vi "Main.vi"() -> ()   [LabVIEW 2016]
uses:
  Type Definitions/Fisher Paykel Motor Profile.ctl
  Type Definitions/FisherPaykel Direction CMD.ctl
  Type Definitions/Fisher Paykel Feedback Commands.ctl
  Type Definitions/Fisher Paykel Agitate Parameters.ctl
  Type Definitions/FisherPaykel Set Sense Profile.ctl
  Type Definitions/Fisher Paykel Friction Profile.ctl
  Type Definitions/Fisher Paykel Bridge Test Profile.ctl
  Trunk/Utility/LabVIEW GEA2 Toolkit v1.0.0.0/type defs/ERD Read Data In.ctl
  Trunk/Utility/LabVIEW GEA2 Toolkit v1.0.0.0/type defs/Data Type.ctl
  Trunk/Washer HCC/Washer HCC NEWFI/Type Definitions/HCC Washer Types.ctl
  Type Definitions/Fisher Paykel Spin PID.ctl
  Trunk/Utility/LabVIEW GEA2 Toolkit v1.0.0.0/type defs/Source_Destination.ctl
  Trunk/Utility/LabVIEW GEA2 Toolkit v1.0.0.0/type defs/Data Out.ctl
  Type Definitions/Fisher Paykel Main Command.ctl
  Trunk/Utility/Save File/File Setup (Public)/Type Definition/Save File DOE LabView Program.ctl
  <vilib>/Utility/file.llb/Write Delimited Spreadsheet (string).vi
  C:/TechLab/NI-2010/Trunk/Utility/LabVIEW GEA2 Toolkit v1.0.0.0/Appliance.NET/GeaCommunication.dll
  Trunk/Utility/LabVIEW GEA2 Toolkit v1.0.0.0/Appliance.NET/GeaCommunication.dll
  Trunk/Utility/LabVIEW GEA2 Toolkit v1.0.0.0/library/GEA2_Toolkit.lvlib
  Trunk/Utility/Save File/File Setup.lvlib
panel:
  out "Exit App":bool
  out "Start DAQ Loop":bool
  in  "OK":bool
  in  "Read ERD List (2017) 2":T1[](array[typedef])=[{"ERD Number"=61623, "Data Type"=enum."string"}, {"ERD Number"=61617, "Data Type"=enum."string"}, {"ERD Number"=65314, "Data Type"=enum."string"}, {"ERD Number"=61563, "Data Type"=enum."string"}, {"ERD Number"=61537, "Data Type"=enum."uint32_t"}, {"ERD Number"=61612, "Data Type"=enum."string"}] {"ERD Number" format="%.0x"}
  out "File  Version":string="Parametric Stand"
  in  "Error In":errorcluster
  out "Error Out":errorcluster
  in  "Tab Control":T3(tab)
  in  "Set Motor Number":bool
  in  "Motor Number":u16=130 max=255 step=1
  in  "Bridge Test Profile":bool
  in  "Move with Bridge Test Profile":T4
  in  "Test Friction Profile":bool
  in  "Move With Friction Test Profile":T5
  in  "Set Sense Profile":bool
  in  "Set Sense Profile":T6
  in  "Move With Stepper Profile":bool
  in  "Reset Fault Flags":bool
  in  "Set Current Limit":bool
  out "Feedback Command Read":string
  out "Agitate Profile Command Read":string
  in  "Send Command":bool
  in  "Stop Motor (Spin)":bool
  in  "Start Agitate Profile":bool
  in  "Agitate Parameters":T7={"Agitate Running Time (sec)"=15, "Direction (CW or CCW)"="1", "RampUpTime (1-600ms)"=250, "TargetSpeed (0-200RPM)"=726, "PlateauTime (0-1800ms 10ms Increment)"=1000, "PauseTime (0-1800ms 10ms Increment)"=600} {"PauseTime (0-1800ms 10ms Increment)" step=10; "PlateauTime (0-1800ms 10ms Increment)" step=10; "TargetSpeed (0-200RPM)" max=1600 step=1; "RampUpTime (1-600ms)" max=600 step=10; "Agitate Running Time (sec)" step=1}
  in  "Start Spin Profile":bool
  out "Spin Profile Command Read":string
  in  "Spin Profile":T9={"Target Speed (RPM)"=23, "Acceleration Rate - (10 Slowest/1000 Fastest)"=10, "Running Time (s)"=0, "Direction (CW or CCW)"="0"} {"Running Time (s)" step=1; "Acceleration Rate - (10 Slowest/1000 Fastest)" min=10 max=1000 step=1; "Target Speed (RPM)" min=23 max=1600 step=1}
  in  "Stop Motor (Agitate)":bool
  in  "Feedback Commands":T10
  in  "Current Limit - (1-50) - (0.1-5A)":u16 max=50 step=1
  in  "Spin PID":T11={"Kp"=1.84, "Ki"=0.03, "Kd"=0.0, "Kc"=0.06} {"Kc" min=0.0 max=1.0; "Kd" min=0.0 max=1.0; "Ki" min=0.0 max=1.0; "Kp" min=0.0 max=16.0}
  in  "Agitate PID":T11={"Kp"=1.84, "Ki"=0.03, "Kd"=0.0, "Kc"=0.06} {"Kc" min=0.0 max=1.0; "Kd" min=0.0 max=1.0; "Ki" min=0.0 max=1.0; "Kp" min=0.0 max=16.0}
  in  "Spin CMD Speed (mS)":u32=150
  in  "Agitate CMD Speed (mS)":u32=150
  in  "Record":bool
  out "File Path":path
  in  "Read Inverter ERDs":bool
  in  "Read Machine ERDs":bool
  out "ERD Array":string[][](array[string])=[["Motor Profile Status (0xF0B7)", "Started"], ["Motor Profile (0xF0B7)", "9"], ["Motor Mode (0xF0B1)", "Idle"], ["Mode Shift Status (0xFF22)", "Agitate State"], ["Sub-Cycle (0xF07B)", "WASH"], ["Remaining Cycle Time(s) (0xF061)", "1707"], ["Target Speed (RPM) (0xF0AC)", "0"], ["Basket Speed (RPM) (0xF0A9)", ""]]
  in  "Read ERD List (2017)":T1[](array[typedef])=[{"ERD Number"=61623, "Data Type"=enum."string"}, {"ERD Number"=61617, "Data Type"=enum."string"}, {"ERD Number"=65314, "Data Type"=enum."string"}, {"ERD Number"=61563, "Data Type"=enum."string"}, {"ERD Number"=61537, "Data Type"=enum."uint32_t"}, {"ERD Number"=61612, "Data Type"=enum."string"}, {"ERD Number"=61609, "Data Type"=enum."uint16_t"}, {"ERD Number"=62218, "Data Type"=enum."string"}, {"ERD Number"=62229, "Data Type"=enum."string"}, {"ERD Number"=62224, "Data Type"=enum."string"}] {"ERD Number" format="%.0x"}
  in  "Run With Machine Controls":bool
  in  "Enable Diagnostic Data":T12=enum."2017 Washer"
  in  "Agitate Parameters Settle Stroke":T7={"Agitate Running Time (sec)"=15, "Direction (CW or CCW)"="1", "RampUpTime (1-600ms)"=250, "TargetSpeed (0-200RPM)"=683, "PlateauTime (0-1800ms 10ms Increment)"=150, "PauseTime (0-1800ms 10ms Increment)"=600} {"PauseTime (0-1800ms 10ms Increment)" step=10; "PlateauTime (0-1800ms 10ms Increment)" step=10; "TargetSpeed (0-200RPM)" max=1600 step=1; "RampUpTime (1-600ms)" max=600 step=10; "Agitate Running Time (sec)" step=1}
  in  "2019 Inverter CMDs":T1[](array[typedef])=[{"ERD Number"=62218, "Data Type"=enum."string"}, {"ERD Number"=62229, "Data Type"=enum."string"}, {"ERD Number"=62224, "Data Type"=enum."string"}] {"ERD Number" format="%.0x"}
  in  "Disable Serial":bool
  out "Use GEA Inverter Output":bool
  in  "GEA Inputs":T13={"Source"=240, "Destination"=35} {"Destination" format="%.0x"; "Source" format="%.0x"}
  out "Debug array":string[](array[string])
  in  "Turn on Text Debug Array":bool
  in  "Inverter Address":T13={"Source"=240, "Destination"=63} {"Destination" format="%.0x"; "Source" format="%.0x"}
  out "Debug Save Array":string[](array[string])
  # "MOTOR CONTROL INTERFACE"
  # "Start Speed > End Speed"
  # "Agitate Profile Parameters"
  # "Agitate Start Parameters"
  # "Spin Profile Parameters"
  # "Spin Start Parameters"
  # "2017 ERD List\nMotor Profile Status (0xF0B7) - string\nMotor Mode (0xF0B1) - string\nMode Shift Status (0xFF22) - string\nSub-Cycle (0xF07B) - string\nRemaining Cycle Time(s) (0xF061) - U32\nTarget Speed (RPM) (0xF0AC) - string\nBasket Speed (0xF0A9) -U16"
  # "2015 ERD List\nMotor Profile Status (0xF319) - string\nMotor Mode (0xF313) - string\nMode Shift Status (0xF31D) - string\nSub-Cycle (0xF213) - string\nRemaining Cycle Time(s) (0xF140) - U32\nTarget Speed (RPM) (0xF30E) - string\nBasket Speed (0xF30B)-U16"
  # "2019 Inverter ERD List\nPower-W (0xF30A) - string\nDriving Speed-RPM (0xF315)-string\nActual Speed-RPM (0xF310)-string"
  # "Agitate Profile Parameters"
  # "Agitate Start Parameters"
  # "Version 34 - Read Machine ERDs and Read Inverter ERDS unchecked by default"
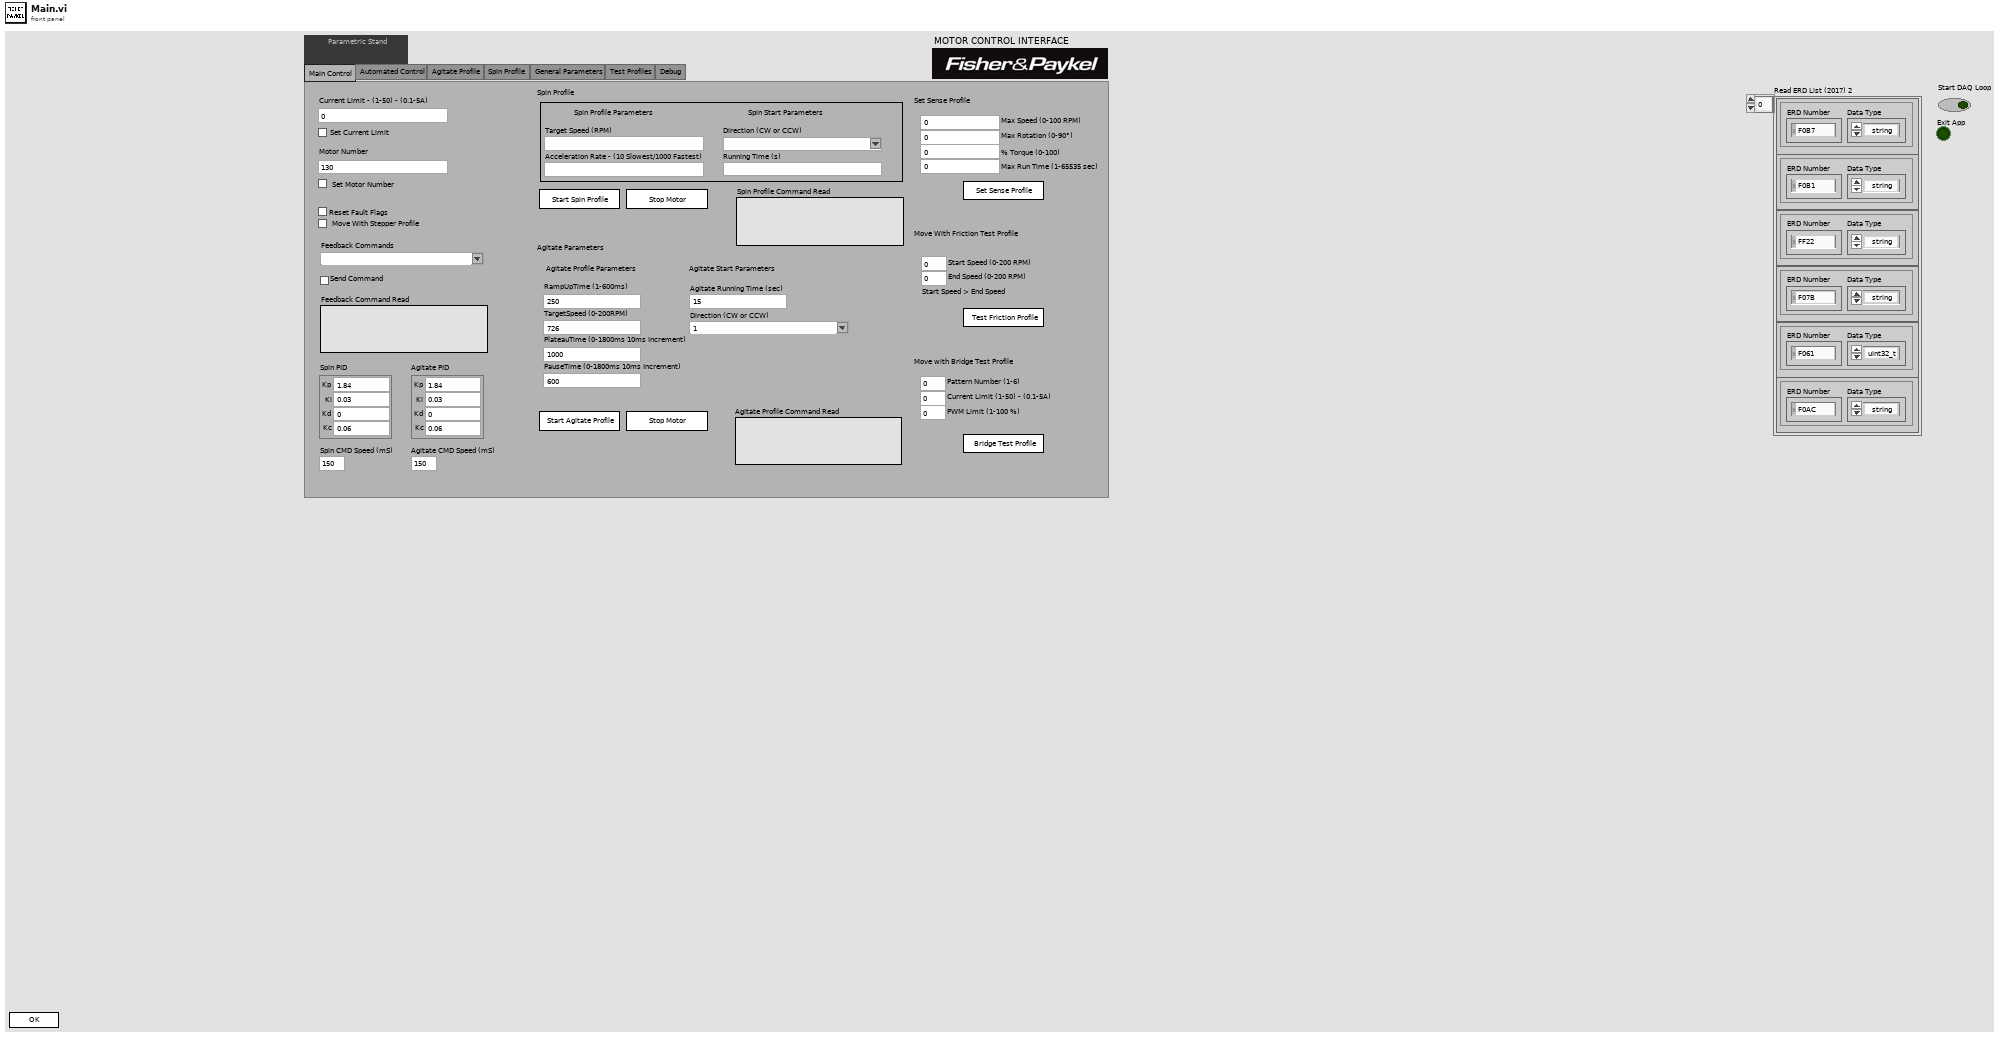
[diagram p1: front panel]
types:
  T1 = typedef "GEA2_Toolkit.lvlib/ERD Read Data In.ctl" = cluster{"ERD Number":u16, "Data Type":T2}
  T2 = typedef "GEA2_Toolkit.lvlib/Data Type.ctl" = enum16{"string", "boolean", "uint8_t", "uint16_t", "uint32_t", "uint64_t"}
  T3 = enum32{"Main Control", "Automated Control", "Agitate Profile", "Spin Profile", "General Parameters", "Test Profiles", "Debug"}
  T4 = typedef "Fisher Paykel Bridge Test Profile.ctl" = cluster{"Pattern Number (1-6)":u16, "Current Limit (1-50) - (0.1-5A)":u16, "PWM Limit (1-100 %)":u16}
  T5 = typedef "Fisher Paykel Friction Profile.ctl" = cluster{"Start Speed (0-200 RPM)":u16, "End Speed (0-200 RPM)":u16}
  T6 = typedef "FisherPaykel Set Sense Profile.ctl" = cluster{"Max Speed (0-100 RPM)":u16, "Max Rotation (0-90°)":u16, "% Torque (0-100)":u16, "Max Run Time (1-65535 sec)":u16}
  T7 = typedef "Fisher Paykel Agitate Parameters.ctl" = cluster{"Agitate Running Time (sec)":u16, "Direction (CW or CCW)":T8, "RampUpTime (1-600ms)":u16, "TargetSpeed (0-200RPM)":u16, "PlateauTime (0-1800ms 10ms Increment)":u16, "PauseTime (0-1800ms 10ms Increment)":u16}
  T8 = typedef "FisherPaykel Direction CMD.ctl" = string
  T9 = typedef "Fisher Paykel Motor Profile.ctl" = cluster{"Target Speed (RPM)":u16, "Acceleration Rate - (10 Slowest/1000 Fastest)":u16, "Running Time (s)":u16, "Direction (CW or CCW)":T8}
  T10 = typedef "Fisher Paykel Feedback Commands.ctl" = string
  T11 = typedef "Fisher Paykel Spin PID.ctl" = cluster{"Kp":dbl, "Ki":dbl, "Kd":dbl, "Kc":dbl}
  T12 = typedef "HCC Washer Types.ctl" = enum16{"", "Viper Washer", "Hawk Washer", "2015 Washer", "2017 Washer"}
  T13 = typedef "GEA2_Toolkit.lvlib/Source_Destination.ctl" = cluster{"Source":u8, "Destination":u8}
  T14 = typedef "Fisher Paykel Main Command.ctl" = string
  T15 = enum32{"invalid app kind", "Development System", "Run Time System", "Student Edition", "Embedded LabVIEW", "Evaluation", "Custom"}
  T16 = enum32{"Invalid", "Standard", "Closed", "Hidden", "Minimized", "Maximized"}
  T17 = typedef "File Setup.lvlib/Save File DOE LabView Program.ctl" = enum16{"No Name Found", "DOE Stand", "Dishwasher Kitchen", "Portable Stand", "HEWH", "Dryer", "Dryer WILT", "HCC", "PRAT", "HEWH RLT", "Refrigeration"}
  T18 = cluster{"Core":cluster{"Current VI Reference":refnum<vi>, "Close Panel on Exit?":bool}, "VISA Output":refnum<visa-resource-name>, "ERD Array":string[][], "Spin Profile":T9, "Agitate Parameters":T7, "GEA Stop Toggle":u8}
  T19 = cluster{"Current VI Reference":refnum<vi>, "Close Panel on Exit?":bool}
  T20 = typedef "FileVersionInformation.ctl" = cluster{"FileVersion":string, "ProductName":string, "InternalName":string, "CompanyName":string, "LegalCopyright":string, "FileDescription":string}
  T21 = enum16{"open", "replace", "create", "open or create", "replace or create", "replace or create with confirmation"}
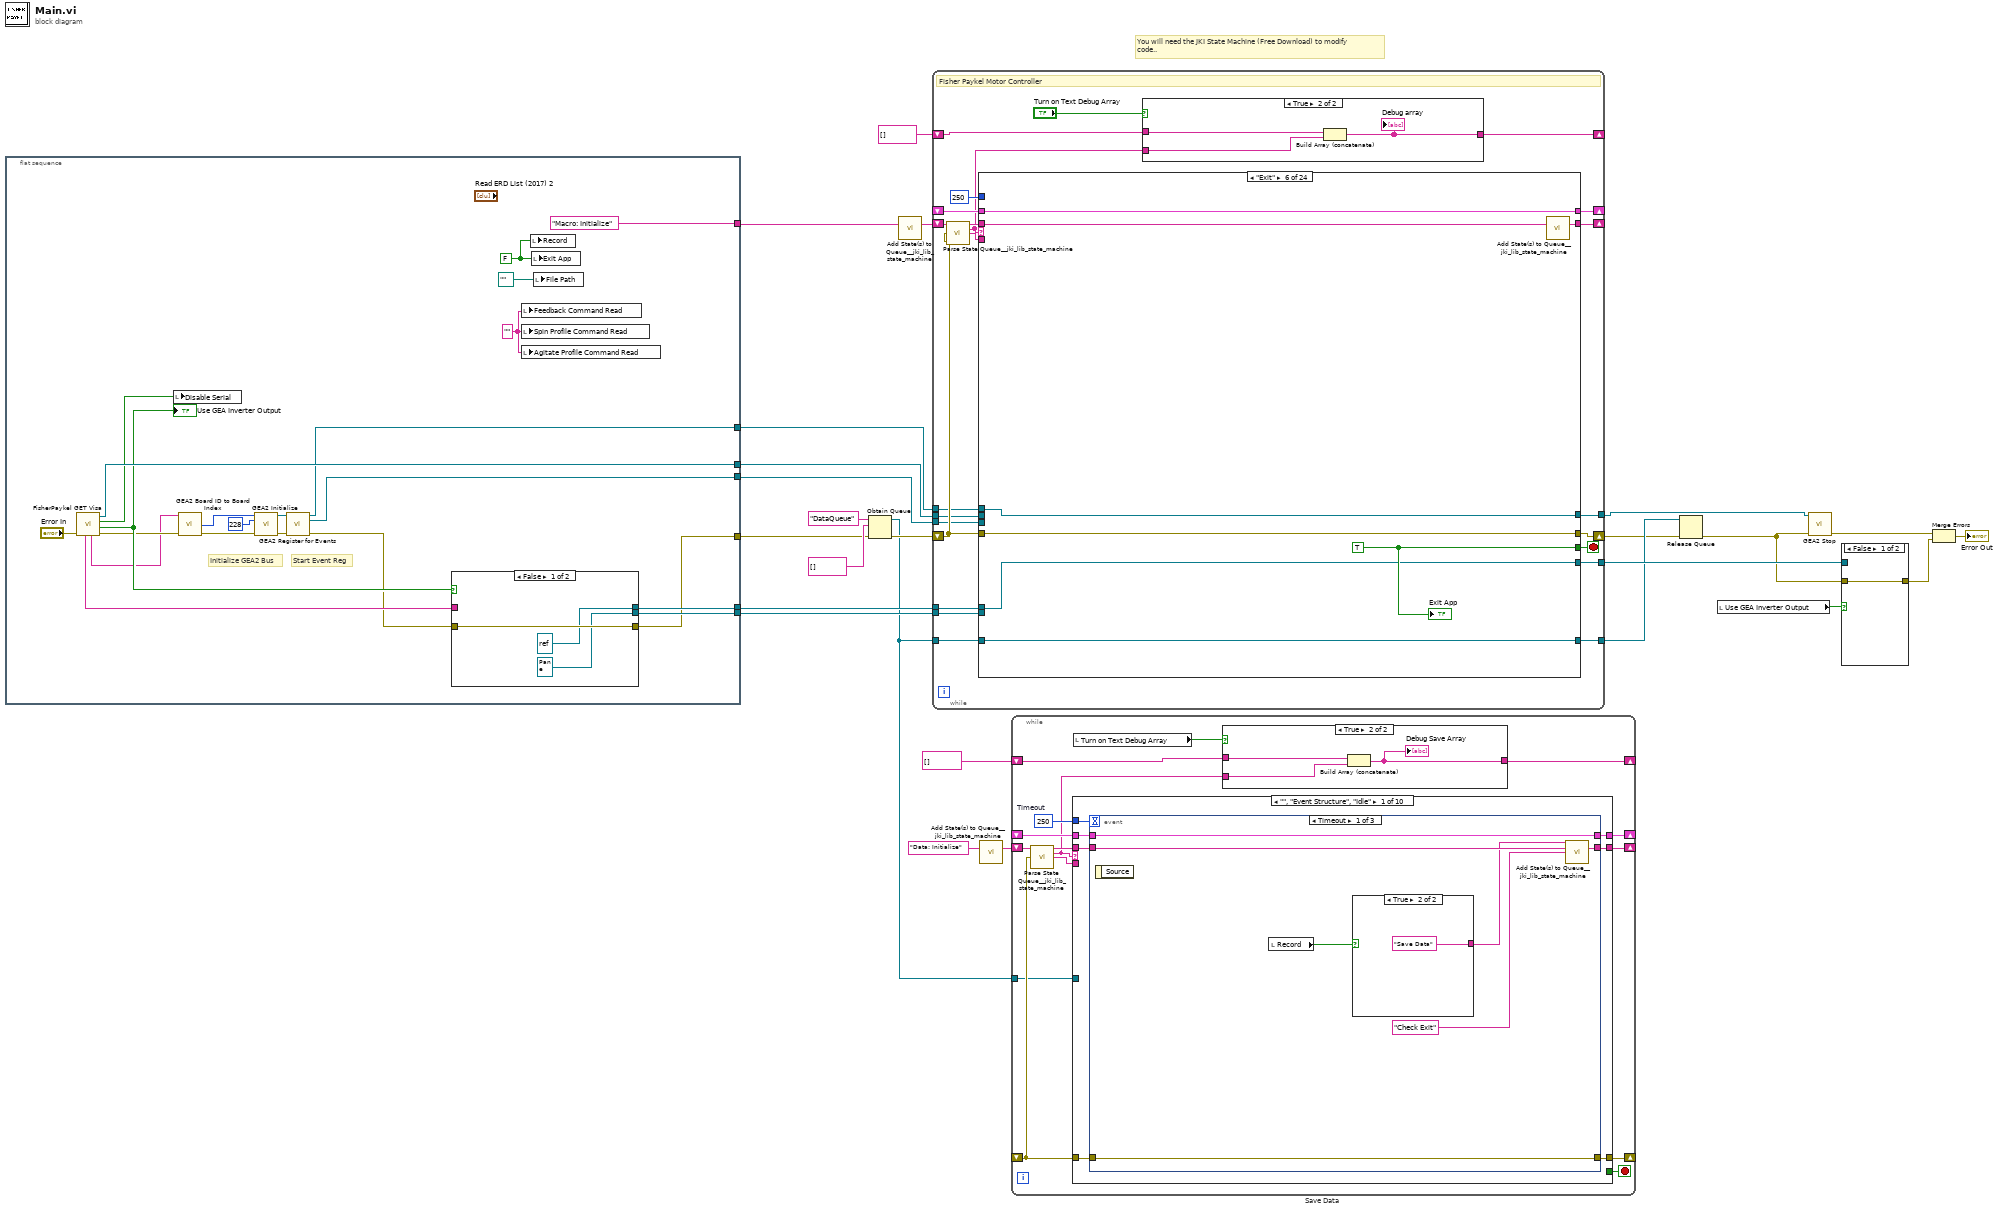
[diagram p0: block diagram]
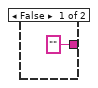
[diagram p3: hidden frame]
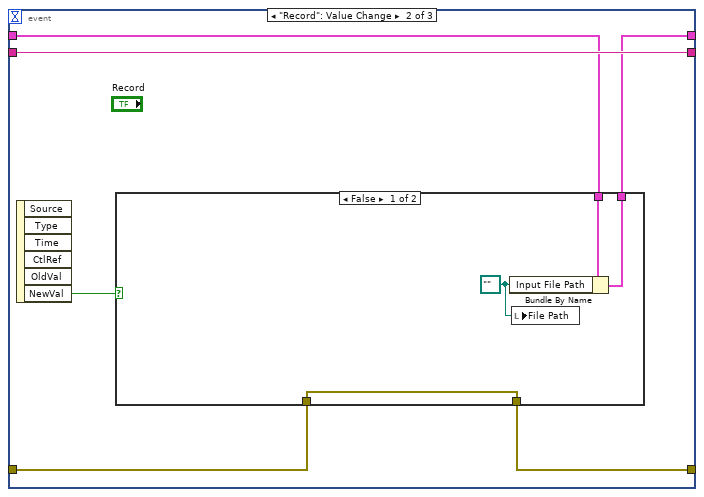
[diagram p4: hidden frame]
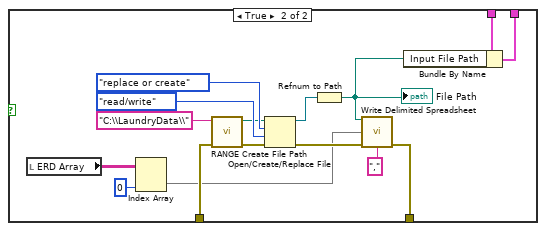
[diagram p5: hidden frame]
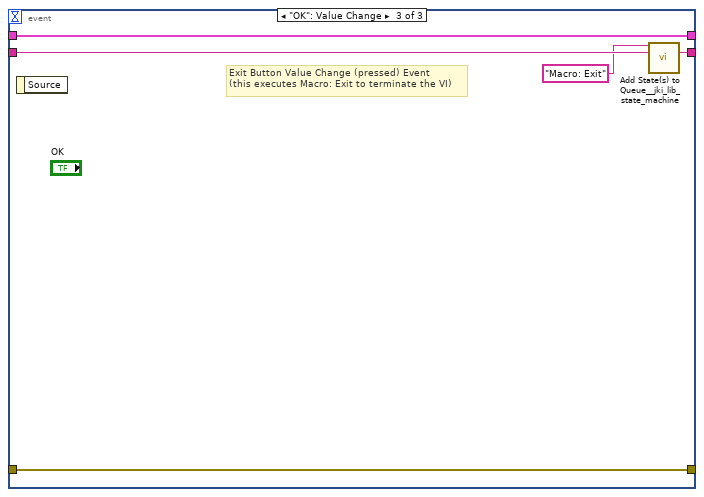
[diagram p6: hidden frame]
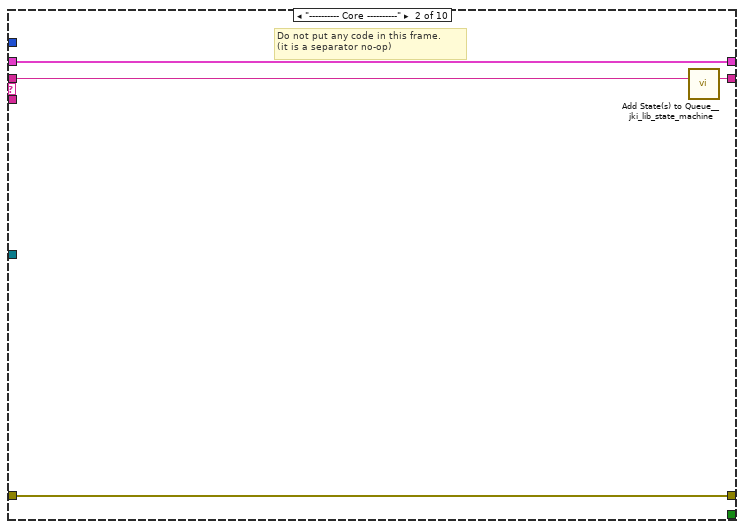
[diagram p7: hidden frame]
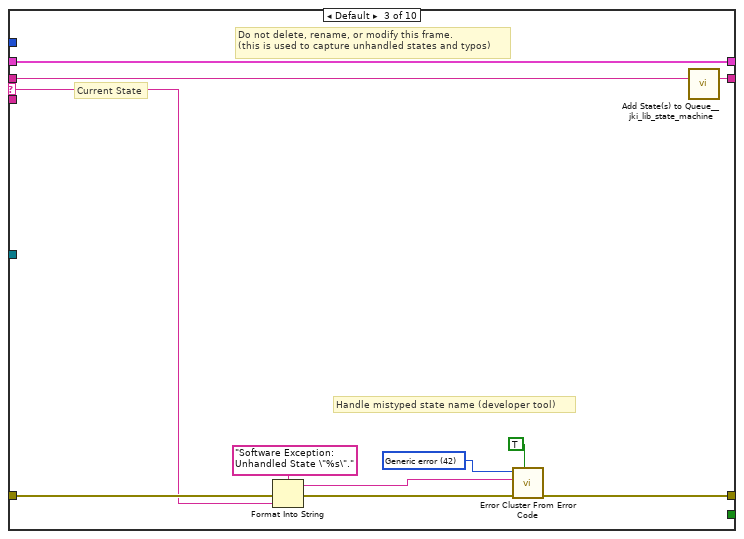
[diagram p8: hidden frame]
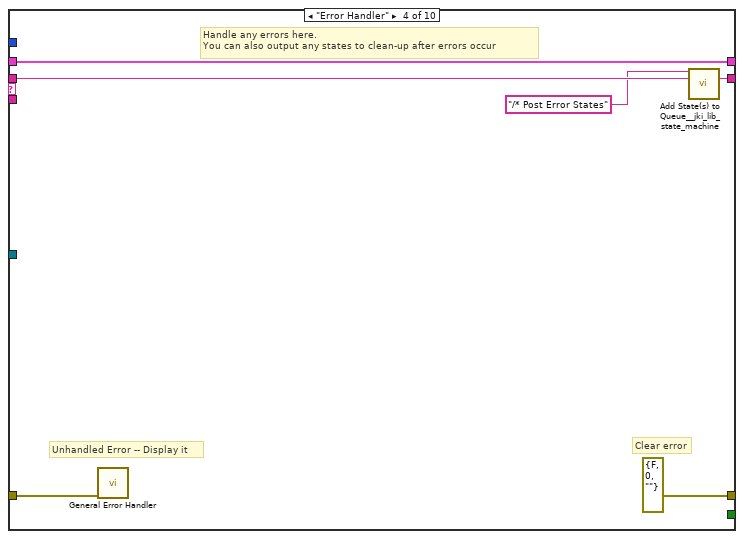
[diagram p9: hidden frame]
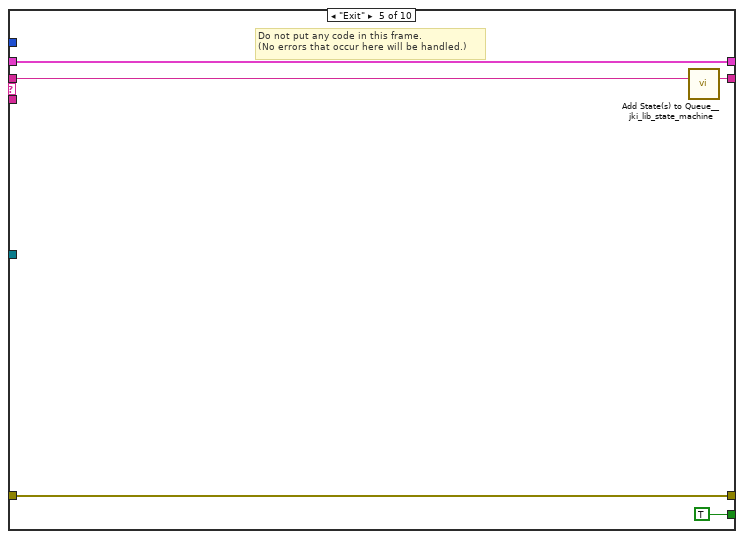
[diagram p10: hidden frame]
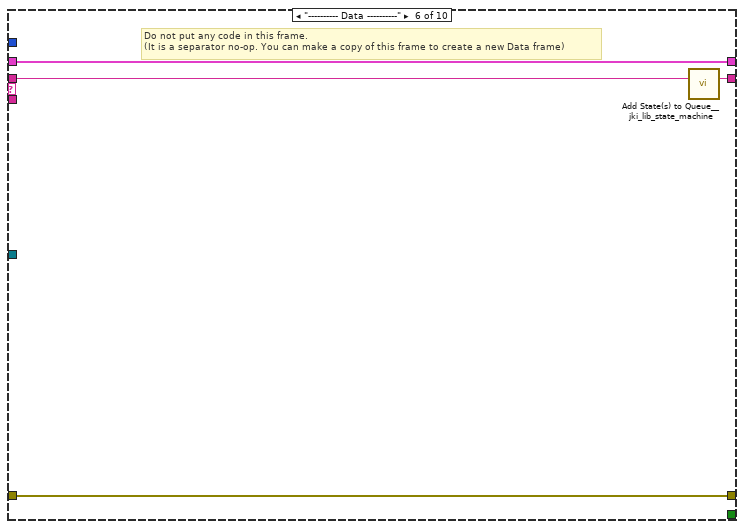
[diagram p11: hidden frame]
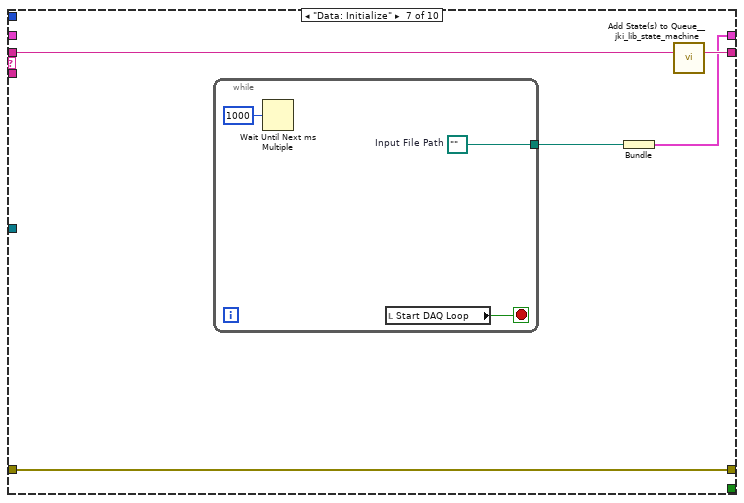
[diagram p12: hidden frame]
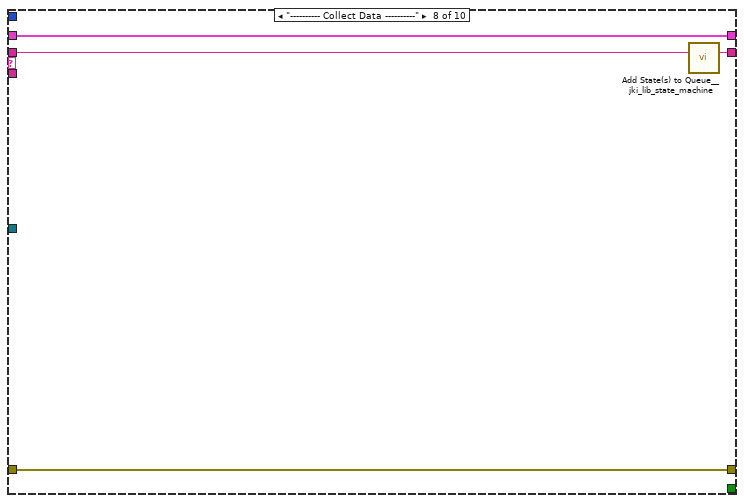
[diagram p13: hidden frame]
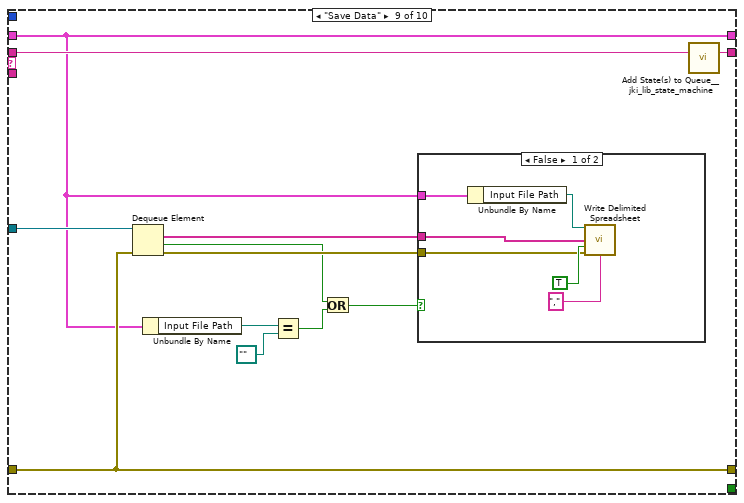
[diagram p14: hidden frame]
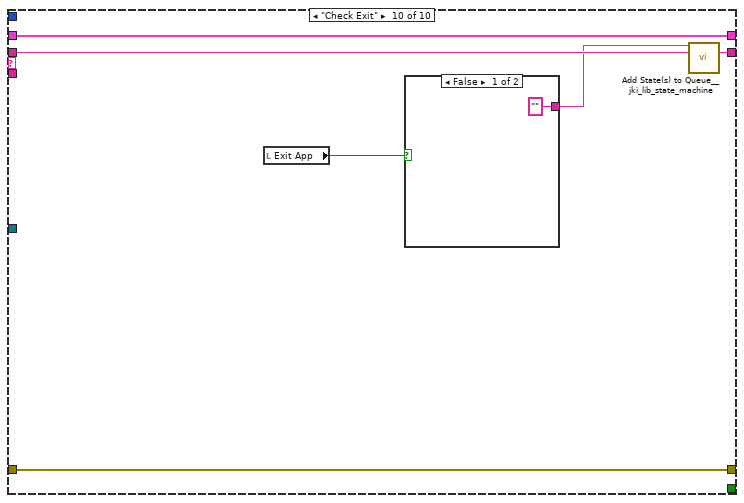
[diagram p16: hidden frame]
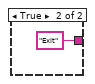
[diagram p17: hidden frame]
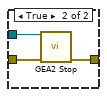
[diagram p18: hidden frame]
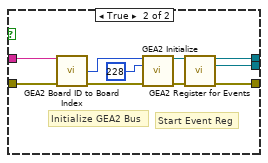
[diagram p19: hidden frame]
diagram:
  # "You will need the JKI State Machine (Free Download) to modify\ncode.."
  n1 = flat-sequence {
    tunnel: ["Macro: Initialize"] -> w24
    tunnel: [w26] -> w1
    tunnel: [w44] -> w23
    tunnel: [w39] -> w22
    tunnel: [w38] -> w21
    tunnel: [w36] -> w18
    tunnel: [w35] -> w17
    frame #0 {
      w28 = FALSE ("Exit App")
      w46 = ""
      # "Start Event Reg"
      # "Initialize GEA2 Bus"
      n2 = call "FisherPaykel GET Visa.vi"("Error In"="Error In") -> ("Error Out"=w33:errorcluster, "Use GEA Inverter Output"=w37:bool, "Disable Serial COM (Debug ONLY) OUT"=w43:bool, "VISA Output"=w44:refnum<visa-resource-name>, "Machine ID Output"=w31:string, "Inverter ID Output"=w34:string)  [unwired: 5 in]
      "Use GEA Inverter Output" <- w37
      n3 = local write "Disable Serial"(w43) -> ()
      n4 = call "GEA2 Board ID to Board Index.vi"("Board ID"=w31, "Error In"=w33) -> ("Board Index"=w30:i32, "Error Out"=w32:errorcluster)  [unwired: 9 in, 3 out]
      n5 = call "GEA2 Initialize.vi"("Board Index"=w30, "Source Address"=u8 228, "error in"=w32) -> ("GEA2 Reference Out"=w40:refnum<k24>, "error out"=w41:errorcluster)  [unwired: 10 in, 1 out]
      n6 = call "GEA2 Register for Events.vi"("GEA2 Reference In"=w40, "Error In"=w41) -> ("GEA2 Reference Out"=w38:refnum<k24>, "GEA2 Event Registration"=w39:refnum<event-registration>, "Error Out"=w27:errorcluster)  [unwired: 11 in]
      n7 = case shown="False" w37 {
        tunnel: w27 -> [w50 w54]
        tunnel: [w50 w57] -> w26
        tunnel: [refnum<k24> refnum ("GEA2 Reference Out") w56] -> w36
        tunnel: [refnum<event-registration> refnum ("GEA2 Event Registration") w55] -> w35
        tunnel: w34 -> [_ w51]
        frame False {
        }
        frame True {
          # "Start Event Reg"
          # "Initialize GEA2 Bus"
          n8 = call "GEA2 Board ID to Board Index.vi"("Board ID"=w51, "Error In"=w54) -> ("Board Index"=w52:i32, "Error Out"=w53:errorcluster)  [unwired: 9 in, 3 out]
          n9 = call "GEA2 Initialize.vi"("Board Index"=w52, "Source Address"=u8 228, "error in"=w53) -> ("GEA2 Reference Out"=w60:refnum<k24>, "error out"=w59:errorcluster)  [unwired: 10 in, 1 out]
          n10 = call "GEA2 Register for Events.vi"("GEA2 Reference In"=w60, "Error In"=w59) -> ("GEA2 Reference Out"=w56:refnum<k24>, "GEA2 Event Registration"=w55:refnum<event-registration>, "Error Out"=w57:errorcluster)  [unwired: 11 in]
        }
      }
      n11 = local write "Feedback Command Read"(w46) -> ()
      n12 = local write "Spin Profile Command Read"(w46) -> ()
      n13 = local write "Agitate Profile Command Read"(w46) -> ()
      n14 = local write "Record"(w28) -> ()
      n15 = local write "Exit App"(w28) -> ()
      n16 = local write "File Path"(path "" ("File Path")) -> ()
    }
  }
  n17 = Obtain Queue(name (unnamed)="DataQueue", element data type=string[] [], error in (no error)=w1) -> (queue out=w6:refnum<queue>, error out=w8:errorcluster)  [unwired: 2 in, 1 out]
  n18 = call <vilib>:"Add State(s) to Queue__jki_lib_state_machine.vi"("State(s) in (\"\")"=w24) -> ("States Out"=w25:string)  [unwired: 14 in]
  n19 = while {
    shift-right: [w77] -> _
    shift-left: _ -> [w76]
    shift-right: [w80] -> w4
    shift-left: w8 -> [w75]
    shift-right: [w79] -> _
    shift-left: w25 -> [w81]
    tunnel: w23 -> [w73]
    tunnel: w22 -> [w72]
    tunnel: w21 -> [w71]
    tunnel: [w70] -> w20
    shift-right: [w68] -> _
    shift-left: string[] [] ("Array") -> [w66]
    tunnel: w18 -> [w65]
    tunnel: w17 -> [w64]
    tunnel: [w63] -> w16
    tunnel: w6 -> [w62]
    tunnel: [w61] -> w5
    stop <- w78 stop-if-true
    # "Fisher Paykel Motor Controller"
    n20 = call <vilib>:"Parse State Queue__jki_lib_state_machine.vi"("State Queue"=w81, "Error In (no error)"=w75) -> ("Remaining States"=w83:string, "Current State"=w69:string, "Arguments"=w82:string)  [unwired: 11 in]
    n21 = case shown="\"Exit\"" w69 {
      selector: w69 -> [_ _ w222 _ _ _ _ _ _ _ _ _ _ _ _ _ _ _ _ _ _ _ _ _]
      tunnel: w83 -> [w97 w218 w226 w247 w256 w264 w271 w290 w314 w325 w337 w346 w361 w390 w398 w411 w418 w429 w465 w523 w539 w560 w580 w600]
      tunnel: w82 -> [_ _ _ _ _ _ _ _ _ _ _ w341 w355 _ _ _ _ _ _ _ _ _ _ _]
      tunnel: w76 -> [w95 w215 w224 w238 w253 w262 w268 _ w310 w322 w334 w344 w357 w387 w395 w408 w415 w427 w460 w520 w532 w546 w572 w594]
      tunnel: [w94 w216 w228 w244 errorcluster {"status"=FALSE, "code"=0, "source"=""} ("error out") w261 w269 w282 w308 w323 w332 w342 w358 w388 w396 w409 w416 w425 w443 w521 w535 w553 w573 w592] -> w80
      tunnel: w75 -> [w93 w216 w227 w244 w252 w261 w269 w283 w311 w323 w335 w343 w359 w388 w396 w409 w416 w426 w463 w521 w536 w554 w574 w593]
      tunnel: [w96 w217 w225 w246 w255 w263 w270 w289 w313 w324 w336 w345 w360 w389 w397 w410 w417 w428 w464 w522 w538 w559 w579 w599] -> w79
      tunnel: [_ _ _ _ _ w260 _ _ _ _ _ _ _ _ _ _ _ _ _ _ _ _ _ _] -> w78
      tunnel: [w92 w215 w224 w245 w253 w262 w268 w288 w310 w322 w334 w344 w357 w387 w395 w408 w415 w427 w459 w520 w531 w545 w572 w594] -> w77
      tunnel: u32 250 ("milliseconds to wait") -> [w91 _ _ _ _ _ _ _ _ _ _ _ _ _ _ _ _ _ _ _ _ _ _ _]
      tunnel: w73 -> [_ _ _ _ _ _ _ w281 _ _ _ _ _ _ _ _ _ _ _ _ _ _ _ _]
      tunnel: w72 -> [_ _ _ _ _ _ _ _ _ _ _ _ _ _ _ _ _ _ w462 _ _ _ _ _]
      tunnel: w71 -> [w90 w214 w221 w235 w250 w259 w267 w276 w304 w321 w331 w340 w354 w386 w393 w401 w414 w421 w461 w519 w526 w541 w562 w582]
      tunnel: [w90 w214 w221 w235 w250 w259 w267 w276 w304 w321 w331 w340 w354 w386 w393 w401 w414 w421 w456 w519 w526 w541 w562 w582] -> w70
      tunnel: w65 -> [w89 w213 w220 w234 w249 w258 w266 w273 w303 w320 w327 w339 w353 w385 w392 w400 w413 w420 w452 w518 w525 w543 w564 w584]
      tunnel: w64 -> [_ _ _ _ _ _ _ _ _ _ _ _ _ _ _ _ _ _ w451 _ _ _ _ _]
      tunnel: [w89 w213 w220 w234 w249 w258 w266 w273 w303 w320 w327 w339 w353 w385 w392 w400 w413 w420 w450 w518 w525 w542 w563 w583] -> w63
      tunnel: w62 -> [w88 w212 w219 w233 w248 w257 w265 w272 w302 w319 w326 w338 w351 w384 w391 w399 w412 w419 w442 w517 w524 w540 w561 w581]
      tunnel: [w88 w212 w219 w233 w248 w257 w265 w272 w302 w319 w326 w338 w351 w384 w391 w399 w412 w419 w437 w517 w524 w540 w561 w581] -> w61
      frame "", "Event Structure", "Idle" {
        n22 = event shown="[14] Panel Close?" {
          selector: _ -> [_ _ _ _ _ _ _ _ _ _ _ _ _ _ _ _]
          dyn-events: _ -> [_ _ _ _ _ _ _ _ _ _ _ _ _ _ _ _]
          timeout: w91 -> [_ _ _ _ _ _ _ _ _ _ _ _ _ _ _ _]
          tunnel: w97 -> [w105 w111 w117 w121 w124 w132 w144 w147 w153 w160 w168 w179 w188 w193 w199 w205]
          tunnel: [w100 w110 w116 w120 w124 w132 w144 w147 w153 w160 w168 w179 w188 w193 w198 w203] -> w96
          tunnel: w95 -> [w103 w112 w114 w122 w125 w133 w143 w148 w152 w161 w169 w180 w186 w192 w196 w202]
          tunnel: [w104 w109 w113 w118 w123 w136 w138 w145 w158 w162 w174 w182 w187 w189 w197 w201] -> w94
          tunnel: w93 -> [w104 w109 w113 w118 w129 w137 w139 w146 w159 w163 w175 w183 w187 w189 w197 w201]
          tunnel: [w103 w112 w114 w122 w125 w133 w143 w148 w152 w161 w169 w180 w185 w191 w196 w202] -> w92
          event Timeout {
            n23 = event-data() -> ()  [unwired: 1 in, 1 out]
            n24 = call <vilib>:"Add State(s) to Queue__jki_lib_state_machine.vi"("State(s) in Front (\"\")"="Read\nGet ERDs" ("State(s) in Front (\"\")"), "State(s) in (\"\")"=w105) -> ("States Out"=w101:string)  [unwired: 13 in]
            n25 = case shown="True" "Run With Machine Controls" {
              tunnel: ["" ("State(s) in Front (\"\")") "Check SubCycle" ("State(s) in Front (\"\")")] -> w99
              frame False {
              }
              frame True {
              }
            }
            n26 = call <vilib>:"Add State(s) to Queue__jki_lib_state_machine.vi"("State(s) in Front (\"\")"=w99, "State(s) in (\"\")"=w101) -> ("States Out"=w100:string)  [unwired: 13 in]
          }
          event "Start Spin Profile": Value Change {
            n27 = event-data() -> ()  [unwired: 1 in, 6 out]
            n28 = call <vilib>:"Add State(s) to Queue__jki_lib_state_machine.vi"("State(s) in Front (\"\")"="Start Spin Profile" ("State(s) in Front (\"\")"), "State(s) in (\"\")"=w111) -> ("States Out"=w110:string)  [unwired: 13 in]
          }
          event "Start Agitate Profile": Value Change {
            n29 = event-data() -> ()  [unwired: 1 in, 6 out]
            n30 = call <vilib>:"Add State(s) to Queue__jki_lib_state_machine.vi"("State(s) in Front (\"\")"="Start Agitate Profile" ("State(s) in Front (\"\")"), "State(s) in (\"\")"=w117) -> ("States Out"=w116:string)  [unwired: 13 in]
          }
          event "Stop Motor (Spin)", "Stop Motor (Agitate)": Value Change {
            n31 = event-data() -> ()  [unwired: 1 in, 6 out]
            n32 = call <vilib>:"Add State(s) to Queue__jki_lib_state_machine.vi"("State(s) in Front (\"\")"="Stop Motor" ("State(s) in Front (\"\")"), "State(s) in (\"\")"=w121) -> ("States Out"=w120:string)  [unwired: 13 in]
          }
          event "Send Command": Value Change {
            n33 = event-data() -> ()  [unwired: 1 in, 6 out]
            n34 = local read "Disable Serial"() -> (w126:bool)
            n35 = Unbundle By Name(w125) -> ("VISA Output"=w128:refnum<visa-resource-name>)
            n36 = call "FisherPaykel Send Command.vi"("Debug"=w126, "error in (no error)"=w129, "Send Command"="Feedback Commands", "VISA Refnum in"=w128) -> ("error out"=w123:errorcluster)  [unwired: 5 in, 2 out]
          }
          event "Set Current Limit": Value Change {
            n37 = event-data() -> ()  [unwired: 1 in, 6 out]
            n38 = local read "Disable Serial"() -> (w135:bool)
            n39 = Unbundle By Name(w133) -> ("VISA Output"=w134:refnum<visa-resource-name>)
            n40 = call "FisherPaykel Set Current Limit.vi"("Debug"=w135, "Error In"=w137, "Current Limit - (1-50) - (0.1-5A)"="Current Limit - (1-50) - (0.1-5A)", "Main Command"=T14 ">ILM", "VISA Refnum in"=w134) -> ("Error Out"=w136:errorcluster)  [unwired: 5 in, 1 out]
          }
          event "Reset Fault Flags": Value Change {
            n41 = event-data() -> ()  [unwired: 1 in, 6 out]
            n42 = local read "Disable Serial"() -> (w140:bool)
            n43 = Unbundle By Name(w143) -> ("VISA Output"=w142:refnum<visa-resource-name>)
            n44 = call "FisherPaykel Send Command.vi"("Debug"=w140, "error in (no error)"=w139, "Send Command"=T14 ">RSF" ("Main Command"), "VISA Refnum in"=w142) -> ("error out"=w138:errorcluster)  [unwired: 5 in, 2 out]
          }
          event "Move With Stepper Profile": Value Change {
            n45 = event-data() -> ()  [unwired: 1 in, 6 out]
            n46 = local read "Disable Serial"() -> (w149:bool)
            n47 = Unbundle By Name(w148) -> ("VISA Output"=w151:refnum<visa-resource-name>)
            n48 = call "FisherPaykel Send Command.vi"("Debug"=w149, "error in (no error)"=w146, "Send Command"=T14 ">GT" ("Main Command"), "VISA Refnum in"=w151) -> ("error out"=w145:errorcluster)  [unwired: 5 in, 2 out]
          }
          event "Set Sense Profile": Value Change {
            n49 = event-data() -> ()  [unwired: 1 in, 6 out]
            n50 = local read "Disable Serial"() -> (w154:bool)
            n51 = Unbundle By Name(w152) -> ("VISA Output"=w155:refnum<visa-resource-name>)
            n52 = call "FisherPaykel Set Sense Profile.vi"("Debug"=w154, "Error In"=w159, "Set Sense Profile"="Set Sense Profile", "Main Command"=T14 ">SNS", "VISA Refnum in"=w155) -> ("Error Out"=w158:errorcluster)  [unwired: 4 in, 2 out]
          }
          event "Test Friction Profile": Value Change {
            n53 = event-data() -> ()  [unwired: 1 in, 6 out]
            n54 = local read "Disable Serial"() -> (w166:bool)
            n55 = Unbundle By Name(w161) -> ("VISA Output"=w165:refnum<visa-resource-name>)
            n56 = call "FisherPaykel Friction Profile.vi"("Debug"=w166, "Error In"=w163, "Move With Friction Test Profile"="Move With Friction Test Profile", "Main Command"=T14 ">GF", "VISA Refnum in"=w165) -> ("Error Out"=w162:errorcluster)  [unwired: 4 in, 2 out]
          }
          event "Bridge Test Profile": Value Change {
            n57 = event-data() -> ()  [unwired: 1 in, 6 out]
            n58 = local read "Disable Serial"() -> (w172:bool)
            n59 = Unbundle By Name(w169) -> ("VISA Output"=w171:refnum<visa-resource-name>)
            n60 = call "FisherPaykel Bridge Profile.vi"("Debug"=w172, "Error In"=w175, "Move with Bridge Test Profile"="Move with Bridge Test Profile", "Main Command"=T14 ">GB", "VISA Refnum in"=w171) -> ("Error Out"=w174:errorcluster)  [unwired: 4 in, 2 out]
          }
          event "Set Motor Number": Value Change {
            n61 = event-data() -> ()  [unwired: 1 in, 6 out]
            n62 = local read "Disable Serial"() -> (w181:bool)
            n63 = Unbundle By Name(w180) -> ("VISA Output"=w178:refnum<visa-resource-name>)
            n64 = call "FisherPaykel Motor Setup 2.vi"("Debug"=w181, "Error In"=w183, "Motor Number"="Motor Number", "Main Command"=T14 ">SMN", "VISA Refnum in"=w178) -> ("Error Out"=w182:errorcluster)  [unwired: 5 in, 1 out]
          }
          event Value Change {
            n65 = event-data() -> ()  [unwired: 1 in, 6 out]
            n66 = local read "Spin Profile"() -> (w184:T9)
            n67 = Bundle By Name(cluster=w186, "Spin Profile"=w184) -> (w185:T18)
          }
          event Value Change {
            n68 = event-data() -> ()  [unwired: 1 in, 6 out]
            n69 = local read "Agitate Parameters"() -> (w190:T7)
            n70 = Bundle By Name(cluster=w192, "Agitate Parameters"=w190) -> (w191:T18)
          }
          event Panel Close? {
            # "Discard the event because we'll close the front panel ourselves in Macro: Exit"
            # "Close Panel button (pressed) Event\n(this executes Macro: Exit to terminate the VI)"
            n71 = event-data() -> ()  [unwired: 1 in, 1 out]
            n72 = event-data("Discard?"=TRUE) -> ()  [unwired: 1 in, 1 out]
            n73 = call <vilib>:"Add State(s) to Queue__jki_lib_state_machine.vi"("State(s) in Front (\"\")"="Macro: Exit", "State(s) in (\"\")"=w199) -> ("States Out"=w198:string)  [unwired: 13 in]
          }
          event Menu Selection (User) {
            n74 = event-data() -> ("ItemTag"=w206:string)  [unwired: 1 in, 6 out]
            n75 = call <vilib>:"Trim Whitespace.vi"("string"="Exit") -> ("trimmed string"=w209:string)  [unwired: 1 in]
            n76 = call <vilib>:"Trim Whitespace.vi"("string"=w206) -> ("trimmed string"=w208:string)  [unwired: 1 in]
            n77 = Equal?(x=w208, y=w209) -> (x = y?=w200:bool)
            n78 = case shown="True" w200 {
              tunnel: ["" "Macro: Exit"] -> w204
              frame False {
              }
              frame True {
              }
            }
            n79 = call <vilib>:"Add State(s) to Queue__jki_lib_state_machine.vi"("State(s) in Front (\"\")"=w204, "State(s) in (\"\")"=w205) -> ("States Out"=w203:string)  [unwired: 13 in]
          }
        }
      }
      frame "---------- Core ----------" {
        n80 = call <vilib>:"Add State(s) to Queue__jki_lib_state_machine.vi"("State(s) in (\"\")"=w218) -> ("States Out"=w217:string)  [unwired: 14 in]
      }
      frame Default {
        w231 = 42 items=["No error", "Argument error", "Memory is full", "Out of zone", "End of file", "File already open", "Generic file I/O error", "File not found", "File permission error", "Disk is full", "Duplicate path", "Too many files open", "System feature not enabled", "Resource file not found", "Cannot add resource", "Resource not found", "Image not found", "Image memory error", "Pen does not exist", "Config type invalid", "Config token not found", "Config parse error", "Config memory error", "Bad external code format", "Bad external code offset", "External code not present", "Null window", "Destroy window error", "Null menu", "Print aborted", "Bad print record", "Print driver error", "Windows error during printing", "Memory error during printing", "Print dialog error", "Generic print error", "Invalid device refnum", "Device not found", "Device parameter error", "Device unit error", "Cannot open device", "Device call aborted", "Generic error", "Cancelled by user", "Object ID too low", "Object ID too high", "Object not in heap", "Unknown heap", "Unknown object (invalid DefProc)", "Unknown object (DefProc not in table)", "Message out of range", "Invalid (null) method", "Unknown message", "Manager call not supported", "Bad address", "Network operation in progress", "Network operation timed out", "Connection is busy", "Network attribute not supported", "Network error", "Address in use", "System out of memory", "Connection aborted", "Connection refused", "Not connected", "Already connected", "Connection closed", "Initialization error (interapplication manager)", "Bad occurrence", "Wait on unbound occurrence handler", "Occurrence queue overflow", "Datalog type conflict", "Unused", "Unrecognized type (interapplication manager)", "Memory corrupt", "Failed to make temporary DLL", "Old CIN version", "Drag socket not found", "Failed to load drop-object", "Failed to register OLE object", "Failed to release OLE object", "Format specifier type mismatch", "Unknown format specifier", "Too few format specifiers", "Too many format specifiers", "Scan failed", "Newer CIN version", "Error converting to variant", "Runtime menu error", "Password tampered", "Variant attribute not found", "Incompatible variant data type", "Event data is not available", "Event Store is not present", "Occurrence is not found", "Event Queue is not created", "Event info is not available", "Refnum passed is NULL", "Error retrieving Class GUID", "Error retrieving CoClass GUID", "Error retrieving TypeLib GUID.", "Bad built application magic bytes.", "Specific driver is different from the specific driver associated with the Logical Name.", "There is no session opened to the class driver.", "Max Error", "MAX - Error with config objects", "MAX - Error loading configuration", "MAX - Group not supported"]
        # "Current State"
        # "Handle mistyped state name (developer tool)"
        n81 = Format Into String(format string="Software Exception: Unhandled State \"%s\"." ("message"), error in=w227, w222) -> (resulting string=w230:string, error out=w229:errorcluster)  [unwired: 1 in]
        n82 = call <vilib>:"Error Cluster From Error Code.vi"("show call chain? (False)"=TRUE, "error in (no error)"=w229, "error message (\"\")"=w230, "error code (0)"=w231) -> ("error out"=w228:errorcluster)  [unwired: 5 in]
        n83 = call <vilib>:"Add State(s) to Queue__jki_lib_state_machine.vi"("State(s) in (\"\")"=w226) -> ("States Out"=w225:string)  [unwired: 14 in]
      }
      frame "Initialize Core Data" {
        # "originally closed?"
        # "exe?"
        # "If panel starts closed or is an EXE, then close it when we exit"
        n84 = property class="VI"() -> ("Front Panel.Open"=w243:bool)  [unwired: 2 in, 2 out]
        n85 = property class="App"() -> ("App.Kind"=w242:T15)  [unwired: 2 in, 2 out]
        n86 = control-ref of="Current VI Reference"() -> (w236:refnum<vi>)
        n87 = Not(x=w243) -> (.not. x?=w240:bool)
        n88 = Equal?(x=w242, y=T15."Run Time System" ("Application:Kind")) -> (x = y?=w239:bool)
        n89 = Or(x=w240, y=w239) -> (x .or. y?=w237:bool)
        n90 = Bundle By Name(cluster=w238, "Core.Current VI Reference"=w236, "Core.Close Panel on Exit?"=w237) -> (w245:T18)
        n91 = call <vilib>:"Add State(s) to Queue__jki_lib_state_machine.vi"("State(s) in (\"\")"=w247) -> ("States Out"=w246:string)  [unwired: 14 in]
      }
      frame "Error Handler" {
        # "Unhandled Error -- Display it"
        # "Clear error"
        n92 = call <vilib>:"General Error Handler.vi"("error in (no error)"=w252) -> ()  [unwired: 10 in, 5 out]
        n93 = call <vilib>:"Add State(s) to Queue__jki_lib_state_machine.vi"("State(s) in Front (\"\")"="/* Post Error States", "State(s) in (\"\")"=w256) -> ("States Out"=w255:string)  [unwired: 13 in]
      }
      frame "Exit" {
        w260 = TRUE
        n94 = call <vilib>:"Add State(s) to Queue__jki_lib_state_machine.vi"("State(s) in (\"\")"=w264) -> ("States Out"=w263:string)  [unwired: 14 in]
        "Exit App" <- w260
      }
      frame "---------- Data ----------" {
        n95 = call <vilib>:"Add State(s) to Queue__jki_lib_state_machine.vi"("State(s) in (\"\")"=w271) -> ("States Out"=w270:string)  [unwired: 14 in]
      }
      frame "Data: Initialize" {
        w274 = u8 1  # GEA Stop Toggle
        w279 = string[][] []  # ERD Array
        w287 = T19 {"Current VI Reference"=refnum, "Close Panel on Exit?"=FALSE}  # Core
        n96 = local read "Use GEA Inverter Output"() -> (w275:bool)
        n97 = case shown="True" w275 {
          tunnel: w281 -> [w298 _]
          tunnel: [w296 ""] -> w280
          frame False {
            n98 = local read "Disable Serial"() -> (w291:bool)
            n99 = Equal?(x=w298, y=refnum<visa-resource-name> refnum) -> (x = y?=w293:bool)
            n100 = Equal?(x=w291, y=FALSE) -> (x = y?=w294:bool)
            n101 = And(x=w294, y=w293) -> (x .and. y?=w292:bool)
            n102 = case shown="False" w292 {
              tunnel: ["" "Macro: Exit"] -> w296
              frame False {
              }
              frame True {
              }
            }
          }
          frame True {
          }
        }
        n103 = Current VI's Path() -> (path=w284:path)
        n104 = call "UTILITY This VIs Path.vi"("path"=w284, "error in (no error)"=w283) -> ("FileVersionInfo Out"=w285:T20, "error out"=w282:errorcluster)  [unwired: 7 in, 5 out]
        n105 = Unbundle By Name(w285) -> ("FileVersion"=→"File  Version":string)
        n106 = Bundle("Core"=w287, "VISA Output"=w281, "ERD Array"=w279, "Spin Profile"="Spin Profile", "Agitate Parameters"="Agitate Parameters", "GEA Stop Toggle"=w274) -> (w288:T18)  [unwired: 1 in]
        n107 = call <vilib>:"Add State(s) to Queue__jki_lib_state_machine.vi"("State(s) in Front (\"\")"=w280, "State(s) in (\"\")"=w290) -> ("States Out"=w289:string)  [unwired: 13 in]
      }
      frame "Data: Cleanup" {
        n108 = Unbundle By Name(w310) -> ("VISA Output"=w305:refnum<visa-resource-name>, "Core.Current VI Reference"=w312:refnum<vi>)
        n109 = Close Reference(reference=w312, error in (no error)=w311) -> (error out=w309:errorcluster)
        n110 = Equal?(x=w305, y=refnum<visa-resource-name> refnum) -> (x = y?=w306:bool)
        n111 = case shown="True" w306 {
          tunnel: w309 -> [w317 w318]
          tunnel: [w316 w318] -> w308
          tunnel: w305 -> [w315 _]
          frame False {
            n112 = VISA Close(VISA resource name=w315, error in (no error)=w317) -> (error out=w316:errorcluster)
          }
          frame True {
          }
        }
        n113 = call <vilib>:"Add State(s) to Queue__jki_lib_state_machine.vi"("State(s) in (\"\")"=w314) -> ("States Out"=w313:string)  [unwired: 14 in]
      }
      frame "---------- UI ----------" {
        n114 = call <vilib>:"Add State(s) to Queue__jki_lib_state_machine.vi"("State(s) in (\"\")"=w325) -> ("States Out"=w324:string)  [unwired: 14 in]
      }
      frame "UI: Initialize" {
        n115 = local read "Use GEA Inverter Output"() -> (w330:bool)
        n116 = local read "Disable Serial"() -> (w329:bool)
        n117 = Unbundle By Name(w334) -> ("VISA Output"=w333:refnum<visa-resource-name>)
        n118 = Or(x=w330, y=w329) -> (x .or. y?=w328:bool)
        n119 = call "FisherPaykel Initialize.vi"("Debug"=w328, "Error In"=w335, "VISA Refnum in"=w333) -> ("Error Out"=w332:errorcluster)  [unwired: 7 in, 1 out]
        n120 = call <vilib>:"Add State(s) to Queue__jki_lib_state_machine.vi"("State(s) in (\"\")"=w337) -> ("States Out"=w336:string)  [unwired: 14 in]
      }
      frame "UI: Cursor Set" {
        # "Argument"
        n121 = case shown="\"Idle\", Default" w341 {
          tunnel: w343 -> [w348 w350]
          tunnel: [w347 w349] -> w342
          frame "Idle", Default {
            n122 = call <vilib>:"Unset Busy.vi"("error in (no error)"=w348) -> ("error out"=w347:errorcluster)  [unwired: 10 in]
          }
          frame "Busy" {
            n123 = call <vilib>:"Set Busy.vi"("error in (no error)"=w350) -> ("error out"=w349:errorcluster)  [unwired: 9 in, 1 out]
          }
        }
        n124 = call <vilib>:"Add State(s) to Queue__jki_lib_state_machine.vi"("State(s) in (\"\")"=w346) -> ("States Out"=w345:string)  [unwired: 14 in]
      }
      frame "UI: Front Panel State" {
        # "Argument"
        n125 = Unbundle By Name(w357) -> ("Core.Current VI Reference"=w356:refnum<vi>)
        n126 = case shown="\"Open\", Default" w355 {
          tunnel: w359 -> [w365 w378]
          tunnel: [w367 w379] -> w358
          tunnel: w356 -> [w366 w376]
          frame "Open", Default {
            n127 = property class="VI"(reference=w366, error in=w365) -> (reference out=w363:refnum<vi>, error out=w364:errorcluster, "Front Panel.Open"=w362:bool)
            n128 = case shown="False" w362 {
              tunnel: [w370 w373] -> w367
              tunnel: w364 -> [w369 w373]
              tunnel: w363 -> [w368 _]
              frame False {
                n129 = invoke class="VI" method="FP.Open"(reference=w368, error in=w369, "Activate"=TRUE, "State"=T16."Standard") -> (error out=w370:errorcluster)  [unwired: 1 in, 4 out]
              }
              frame True {
              }
            }
          }
          frame "Close" {
            n130 = property class="VI"(reference=w376, error in=w378) -> (reference out=w375:refnum<vi>, error out=w377:errorcluster, "Front Panel.Open"=w374:bool)
            n131 = case shown="True" w374 {
              tunnel: [w380 w383] -> w379
              tunnel: w377 -> [w380 w382]
              tunnel: w375 -> [_ w381]
              frame False {
              }
              frame True {
                n132 = invoke class="VI" method="FP.Close"(reference=w381, error in=w382) -> (error out=w383:errorcluster)  [unwired: 1 in, 2 out]
              }
            }
          }
        }
        n133 = call <vilib>:"Add State(s) to Queue__jki_lib_state_machine.vi"("State(s) in (\"\")"=w361) -> ("States Out"=w360:string)  [unwired: 14 in]
        "Start DAQ Loop" <- TRUE ("Start DAQ Loop")
      }
      frame "---------- Macro ----------" {
        n134 = call <vilib>:"Add State(s) to Queue__jki_lib_state_machine.vi"("State(s) in (\"\")"=w390) -> ("States Out"=w389:string)  [unwired: 14 in]
      }
      frame "Macro: Initialize" {
        w394 = "Data: Initialize\nInitialize Core Data\nUI: Initialize\nUI: Front Panel State >> Open"  # Data: Initialize Initialize Core Data UI: Initialize UI: Front Panel State >> Open
        n135 = call <vilib>:"Add State(s) to Queue__jki_lib_state_machine.vi"("State(s) in Front (\"\")"=w394, "State(s) in (\"\")"=w398) -> ("States Out"=w397:string)  [unwired: 13 in]
      }
      frame "Macro: Exit" {
        # "Exit Macro\n(This is called once, when the VI exits)"
        n136 = Unbundle By Name(w408) -> ("Core.Close Panel on Exit?"=w407:bool)
        n137 = Select(t="UI: Front Panel State >> Close", s=w407, f="") -> (s? t:f=w404:string)
        n138 = call <vilib>:"Add State(s) to Queue__jki_lib_state_machine.vi"("State(s) in (\"\")"=w404, "State(s) at Back (\"\")"="Data: Cleanup\nExit") -> ("States Out"=w402:string)  [unwired: 13 in]
        n139 = call <vilib>:"Add State(s) to Queue__jki_lib_state_machine.vi"("State(s) in Front (\"\")"=w402, "State(s) in (\"\")"=w411) -> ("States Out"=w410:string)  [unwired: 13 in]
      }
      frame "---------- Data Collection ----------" {
        n140 = call <vilib>:"Add State(s) to Queue__jki_lib_state_machine.vi"("State(s) in (\"\")"=w418) -> ("States Out"=w417:string)  [unwired: 14 in]
      }
      frame "Read" {
        n141 = local read "Feedback Commands"() -> (w424:T10)
        n142 = Equal?(x=w424, y=T10 "") -> (x = y?=w422:bool)
        n143 = case shown="True" w422 {
          tunnel: w427 -> [w435 _]
          tunnel: w426 -> [w432 w436]
          tunnel: [w431 w436] -> w425
          frame False {
            n144 = local read "Disable Serial"() -> (w433:bool)
            n145 = Unbundle By Name(w435) -> ("VISA Output"=w434:refnum<visa-resource-name>)
            n146 = call "FisherPaykel Read Serial Command.vi"("Debug"=w433, "Error In"=w432, "VISA Refnum in"=w434) -> ("Error Out"=w431:errorcluster, "Serial Read Command"=→"Feedback Command Read":string)  [unwired: 6 in, 1 out]
          }
          frame True {
          }
        }
        n147 = call <vilib>:"Add State(s) to Queue__jki_lib_state_machine.vi"("State(s) in (\"\")"=w429) -> ("States Out"=w428:string)  [unwired: 14 in]
      }
      frame "Get ERDs" {
        # "Get the ERDs. This needs cleaned\nup. I was lazy when 2015 ERDs all changed"
        n148 = case shown="False" "Read Machine ERDs" {
          tunnel: w463 -> [w476 w490]
          tunnel: w462 -> [w475 w489]
          tunnel: w461 -> [w474 w488]
          tunnel: [w476 w480] -> w458
          tunnel: [w475 w479] -> w457
          tunnel: [w474 w478] -> w455
          tunnel: [string[][] [] ("ERD Array") w477] -> w454
          frame False {
          }
          frame True {
            n149 = call "GEA2 Collect HEWH ERDs.vi"(".NET Refnum in"=w488, "GEA Inputs"="GEA Inputs", "GEA2 Event Registration In"=w489, "Disable ERD (Main)"=FALSE, "error in (no error)"=w490, "Custom ERDs"=TRUE, "Disable ERD Filter"=TRUE, "LV Program"=Save_File_DOE_LabView_Program."DOE Stand", "Read ERD List"="Read ERD List (2017)", "Enable Diagnostic Data"="Enable Diagnostic Data") -> (".NET Refnum out"=w478:refnum<k24>, "GEA2 Event Registration Out"=w479:refnum<event-registration>, "ERD Array"=w477:string[][], "error out"=w480:errorcluster)  [unwired: 4 in, 2 out]
          }
        }
        n150 = local read "Use GEA Inverter Output"() -> (w453:bool)
        n151 = case shown="False" w453 {
          tunnel: w458 -> [w492 w503]
          tunnel: w457 -> [_ _]
          tunnel: [w492 w502] -> w444
          tunnel: [w494 w499] -> w456
          tunnel: w455 -> [w494 w499]
          tunnel: w454 -> [w493 w501]
          tunnel: [w493 w500] -> w448
          tunnel: w452 -> [w491 w498]
          tunnel: w451 -> [_ w497]
          tunnel: [w491 w496] -> w450
          tunnel: "Read Inverter ERDs" -> [_ w495]
          frame False {
          }
          frame True {
            n152 = case shown="True" w495 {
              tunnel: w503 -> [w505 w514]
              tunnel: [w505 w513] -> w502
              tunnel: w501 -> [w506 w511]
              tunnel: [w506 w510] -> w500
              tunnel: w498 -> [w504 w509]
              tunnel: w497 -> [_ w508]
              tunnel: [w504 w507] -> w496
              frame False {
              }
              frame True {
                n153 = local read "Inverter Address"() -> (w516:T13)
                n154 = call "GEA2 FP ERDs.vi"("2019 Inverter CMDs"="2019 Inverter CMDs", "Inverter Address"=w516, "Error In"=w514, "GEA2 Event Registration In"=w508, ".NET Refnum in"=w509) -> ("Error Out"=w513:errorcluster, "Data"=w512:string[][], ".NET Refnum out"=w507:refnum<k24>)  [unwired: 2 in, 2 out]
                n155 = Build Array (concatenate)(w511, w512) -> (w510:string[][])
              }
            }
          }
        }
        n156 = call "UTILITY E-Time.vi"() -> ("Elapsed Time (sec)"=w449:dbl)  [unwired: 9 in, 2 out]
        n157 = call "UTILITY General Time Header.vi"("Elapsed Time"=w449) -> ("Total Array"=w447:string[][])  [unwired: 9 in, 1 out]
        n158 = local read "Record"() -> (w438:bool)
        n159 = Build Array (concatenate)(w447, w448) -> (w441:string[][])
        "ERD Array" <- w441
        n160 = Index Array(array=w441, index (col)=1 ("disabled index (col)")) -> (element=w439:string[])  [unwired: 1 in]
        n161 = Bundle By Name(cluster=w460, "ERD Array"=w441) -> (w459:T18)
        n162 = case shown="True" w438 {
          tunnel: w444 -> [w467 w472]
          tunnel: [w467 w471] -> w443
          tunnel: w442 -> [w466 w470]
          tunnel: w439 -> [_ w469]
          tunnel: [w466 w468] -> w437
          frame False {
          }
          frame True {
            n163 = Enqueue Element(queue=w470, element=w469, error in (no error)=w472) -> (queue out=w468:refnum<queue>, error out=w471:errorcluster)  [unwired: 1 in, 1 out]
          }
        }
        n164 = call <vilib>:"Add State(s) to Queue__jki_lib_state_machine.vi"("State(s) in (\"\")"=w465) -> ("States Out"=w464:string)  [unwired: 14 in]
      }
      frame "-------- Motor Control --------" {
        n165 = call <vilib>:"Add State(s) to Queue__jki_lib_state_machine.vi"("State(s) in (\"\")"=w523) -> ("States Out"=w522:string)  [unwired: 14 in]
      }
      frame "Check SubCycle" {
        n166 = local read "Agitate Parameters"() -> (w527:T7)
        n167 = Unbundle By Name(w532) -> ("ERD Array"=w537:string[][], "Spin Profile"=w533:T9)
        n168 = call "FisherPaykel Check SubCycle.vi"("Agitate Parameters Settle Stroke"="Agitate Parameters Settle Stroke", "Error In"=w536, "Agitate Parameters"=w527, "Spin Profile"=w533, "ERD Array"=w537) -> ("Error Out"=w535:errorcluster, "Agitate Parameters Output"=w529:T7, "Spin Profile Output"=w530:T9, "States Output"=w534:string)  [unwired: 3 in]
        n169 = Bundle By Name(cluster=w532, "Spin Profile"=w530, "Agitate Parameters"=w529) -> (w531:T18)
        n170 = call <vilib>:"Add State(s) to Queue__jki_lib_state_machine.vi"("State(s) in Front (\"\")"=w534, "State(s) in (\"\")"=w539) -> ("States Out"=w538:string)  [unwired: 13 in]
      }
      frame "Stop Motor" {
        n171 = Unbundle By Name(w546) -> ("VISA Output"=w552:refnum<visa-resource-name>, "GEA Stop Toggle"=w547:u8)
        n172 = local read "Use GEA Inverter Output"() -> (w549:bool)
        n173 = local read "Disable Serial"() -> (w551:bool)
        n174 = call "FisherPaykel Stop Motor.vi"("VISA Refnum in"=w552, "Debug"=w551, "Use GEA Inverter Output"=w549, "Main Command"=T14 ">STP", "GEA2 Reference In"=w543, "Error In"=w554, "GEA Stop Toggle"=w547, "GEA Inputs"="Inverter Address") -> ("VISA Refnum out"=w556:refnum<visa-resource-name>, "GEA2 Reference Out"=w542:refnum<k24>, "GEA Stop Toggle Out"=w544:u8, "Error Out"=w557:errorcluster)  [unwired: 3 in, 1 out]
        n175 = Or(x=w549, y=w551) -> (x .or. y?=w550:bool)
        n176 = call "FisherPaykel Read Serial Command.vi"("Debug"=w550, "Error In"=w557, "VISA Refnum in"=w556) -> ("Error Out"=w553:errorcluster, "Serial Read Command"=w555:string)  [unwired: 6 in, 1 out]
        n177 = local write "Agitate Profile Command Read"(w555) -> ()
        n178 = local write "Spin Profile Command Read"(w555) -> ()
        n179 = Bundle By Name(cluster=w546, "GEA Stop Toggle"=w544) -> (w545:T18)
        n180 = call <vilib>:"Add State(s) to Queue__jki_lib_state_machine.vi"("State(s) in (\"\")"=w560) -> ("States Out"=w559:string)  [unwired: 14 in]
      }
      frame "Start Spin Profile" {
        n181 = local read "Use GEA Inverter Output"() -> (w566:bool)
        n182 = local read "Inverter Address"() -> (w565:T13)
        n183 = Unbundle By Name(w572) -> ("VISA Output"=w577:refnum<visa-resource-name>, "Spin Profile"=w571:T9)
        n184 = call "FisherPaykel Spin State.vi"("VISA Refnum in"=w577, "Debug"="Disable Serial", "Use GEA Inverter Output"=w566, "Spin Profile"=w571, "GEA2 Reference In"=w564, "error in (no error)"=w574, "PID"="Spin PID", "Agitate CMD Speed"="Spin CMD Speed (mS)", "GEA Inputs"=w565) -> ("VISA Refnum out"=w575:refnum<visa-resource-name>, "GEA2 Reference Out"=w563:refnum<k24>, "error out"=w576:errorcluster)  [unwired: 4 in]
        n185 = Or(x=w566, y="Disable Serial") -> (x .or. y?=w569:bool)
        n186 = call "FisherPaykel Read Serial Command.vi"("Debug"=w569, "Error In"=w576, "VISA Refnum in"=w575) -> ("Error Out"=w573:errorcluster, "Serial Read Command"=→"Spin Profile Command Read":string)  [unwired: 6 in, 1 out]
        n187 = call <vilib>:"Add State(s) to Queue__jki_lib_state_machine.vi"("State(s) in (\"\")"=w580) -> ("States Out"=w579:string)  [unwired: 14 in]
      }
      frame "Start Agitate Profile" {
        n188 = local read "Use GEA Inverter Output"() -> (w586:bool)
        n189 = Unbundle By Name(w594) -> ("VISA Output"=w596:refnum<visa-resource-name>, "Agitate Parameters"=w591:T7)
        n190 = local read "Inverter Address"() -> (w585:T13)
        n191 = local read "Disable Serial"() -> (w589:bool)
        n192 = call "FisherPaykel Agitate State.vi"("VISA Refnum in"=w596, "Debug"=w589, "Use GEA Inverter Output"=w586, "Agitate Parameters"=w591, "GEA2 Reference In"=w584, "Error In"=w593, "Agitate PID"="Agitate PID", "Agitate CMD Speed"="Agitate CMD Speed (mS)", "GEA Inputs"=w585) -> ("VISA resource name out"=w597:refnum<visa-resource-name>, "GEA2 Reference Out"=w583:refnum<k24>, "Error Out"=w598:errorcluster)  [unwired: 4 in]
        n193 = Or(x=w586, y=w589) -> (x .or. y?=w588:bool)
        n194 = call "FisherPaykel Read Serial Command.vi"("Debug"=w588, "Error In"=w598, "VISA Refnum in"=w597) -> ("Error Out"=w592:errorcluster, "Serial Read Command"=→"Agitate Profile Command Read":string)  [unwired: 6 in, 1 out]
        n195 = call <vilib>:"Add State(s) to Queue__jki_lib_state_machine.vi"("State(s) in (\"\")"=w600) -> ("States Out"=w599:string)  [unwired: 14 in]
      }
    }
    n196 = case shown="True" "Turn on Text Debug Array" {
      tunnel: w69 -> [_ w87]
      tunnel: [w84 w86] -> w68
      tunnel: w66 -> [w84 w85]
      frame False {
      }
      frame True {
        n197 = Build Array (concatenate)(w85, w87) -> (w86:string[])
        "Debug array" <- w86
      }
    }
  }
  n198 = call <vilib>:"Add State(s) to Queue__jki_lib_state_machine.vi"("State(s) in (\"\")"="Data: Initialize") -> ("States Out"=w11:string)  [unwired: 14 in]
  n199 = while "Save Data" {
    shift-right: [w609] -> _
    shift-left: _ -> [w608]
    shift-right: [w612] -> _
    shift-left: _ -> [w606]
    shift-right: [w611] -> _
    shift-left: w11 -> [w613]
    tunnel: w6 -> [w605]
    shift-right: [w603] -> _
    shift-left: string[] [] ("Array") -> [w604]
    stop <- w610 stop-if-true
    w607 = 250  # Timeout
    n200 = call <vilib>:"Parse State Queue__jki_lib_state_machine.vi"("State Queue"=w613, "Error In (no error)"=w606) -> ("Remaining States"=w615:string, "Current State"=w602:string, "Arguments"=w614:string)  [unwired: 11 in]
    n201 = case shown="\"\", \"Event Structure\", \"Idle\"" w602 {
      selector: w602 -> [_ _ w671 _ _ _ _ _ _ _]
      tunnel: w615 -> [w626 w670 w675 w687 w692 w696 w701 w708 w720 w732]
      tunnel: w614 -> [_ _ _ _ _ _ _ _ _ _]
      tunnel: w608 -> [w624 w667 w673 w684 w690 w693 _ w705 w712 w729]
      tunnel: [w623 w668 w677 errorcluster {"status"=FALSE, "code"=0, "source"=""} ("error out") w689 w694 w698 w706 w717 w730] -> w612
      tunnel: w606 -> [w622 w668 w676 w683 w689 w694 w698 w706 w717 w730]
      tunnel: [w625 w669 w674 w686 w691 w695 w700 w707 w719 w731] -> w611
      tunnel: [_ _ _ _ TRUE _ _ _ _ _] -> w610
      tunnel: [w621 w667 w673 w684 w690 w693 w699 w705 w712 w729] -> w609
      tunnel: w607 -> [w620 _ _ _ _ _ _ _ _ _]
      tunnel: w605 -> [_ _ _ _ _ _ _ _ w718 _]
      frame "", "Event Structure", "Idle" {
        n202 = event shown="[0] Timeout" {
          selector: _ -> [_ _ _]
          dyn-events: _ -> [_ _ _]
          timeout: w620 -> [_ _ _]
          tunnel: w626 -> [w633 w641 w666]
          tunnel: [w632 w641 w665] -> w625
          tunnel: w624 -> [w630 w638 w663]
          tunnel: [w631 w639 w664] -> w623
          tunnel: w622 -> [w631 w640 w664]
          tunnel: [w630 w637 w663] -> w621
          event Timeout {
            n203 = event-data() -> ()  [unwired: 1 in, 1 out]
            n204 = local read "Record"() -> (w628:bool)
            n205 = case shown="True" w628 {
              tunnel: ["" ("State(s) in Front (\"\")") "Save Data" ("State(s) in Front (\"\")")] -> w629
              frame False {
              }
              frame True {
              }
            }
            n206 = call <vilib>:"Add State(s) to Queue__jki_lib_state_machine.vi"("State(s) in Front (\"\")"=w629, "State(s) in (\"\")"=w633, "State(s) at Back (\"\")"="Check Exit" ("State(s) at Back (\"\")")) -> ("States Out"=w632:string)  [unwired: 12 in]
          }
          event "Record": Value Change {
            n207 = event-data() -> ("NewVal"=w636:bool)  [unwired: 1 in, 5 out]
            n208 = case shown="False" w636 {
              tunnel: w640 -> [w645 w654]
              tunnel: [w645 w652] -> w639
              tunnel: w638 -> [w644 w648]
              tunnel: [w643 w647] -> w637
              frame False {
                w642 = path "" ("Input File Path")
                n209 = Bundle By Name(cluster=w644, "Input File Path"=w642) -> (w643:cluster{"Input File Path":path})
                n210 = local write "File Path"(w642) -> ()
              }
              frame True {
                n211 = local read "ERD Array"() -> (w651:string[][])
                n212 = Index Array(array=w651, index (col)=0 ("disabled index (col)")) -> (element=w650:string[])  [unwired: 1 in]
                n213 = call "RANGE Create File Path.vi"("Error In"=w654, "File Path"="C:\\LaundryData\\") -> ("Error Out"=w656:errorcluster, "Path"=w658:path)  [unwired: 8 in]
                n214 = Open/Create/Replace File(file path (use dialog)=w658, error in=w656, operation (0:open)=T21."replace or create", access (0:read/write)=enum16{"read/write", "read-only", "write-only"}."read/write") -> (refnum out=w657:refnum<file>, error out=w653:errorcluster)  [unwired: 2 in, 1 out]
                n215 = Refnum to Path(1:w657) -> (0:w646:path)
                "File Path" <- w646
                n216 = call-poly <vilib>:"Write Delimited Spreadsheet.vi"("file path (dialog if empty)"=w646, "1D data"=w650, "error in (no error)"=w653, "delimiter (\\t)"="," ("delimiter (\\t)")) -> ("error out"=w652:errorcluster)  [unwired: 10 in, 1 out]
                n217 = Bundle By Name(cluster=w648, "Input File Path"=w646) -> (w647:cluster{"Input File Path":path})
              }
            }
          }
          event "OK": Value Change {
            # "Exit Button Value Change (pressed) Event\n(this executes Macro: Exit to terminate the VI)"
            n218 = event-data() -> ()  [unwired: 1 in, 1 out]
            n219 = call <vilib>:"Add State(s) to Queue__jki_lib_state_machine.vi"("State(s) in Front (\"\")"="Macro: Exit", "State(s) in (\"\")"=w666) -> ("States Out"=w665:string)  [unwired: 13 in]
          }
        }
      }
      frame "---------- Core ----------" {
        # "Do not put any code in this frame.\n(it is a separator no-op)"
        n220 = call <vilib>:"Add State(s) to Queue__jki_lib_state_machine.vi"("State(s) in (\"\")"=w670) -> ("States Out"=w669:string)  [unwired: 14 in]
      }
      frame Default {
        w680 = 42 items=["No error", "Argument error", "Memory is full", "Out of zone", "End of file", "File already open", "Generic file I/O error", "File not found", "File permission error", "Disk is full", "Duplicate path", "Too many files open", "System feature not enabled", "Resource file not found", "Cannot add resource", "Resource not found", "Image not found", "Image memory error", "Pen does not exist", "Config type invalid", "Config token not found", "Config parse error", "Config memory error", "Bad external code format", "Bad external code offset", "External code not present", "Null window", "Destroy window error", "Null menu", "Print aborted", "Bad print record", "Print driver error", "Windows error during printing", "Memory error during printing", "Print dialog error", "Generic print error", "Invalid device refnum", "Device not found", "Device parameter error", "Device unit error", "Cannot open device", "Device call aborted", "Generic error", "Cancelled by user", "Object ID too low", "Object ID too high", "Object not in heap", "Unknown heap", "Unknown object (invalid DefProc)", "Unknown object (DefProc not in table)", "Message out of range", "Invalid (null) method", "Unknown message", "Manager call not supported", "Bad address", "Network operation in progress", "Network operation timed out", "Connection is busy", "Network attribute not supported", "Network error", "Address in use", "System out of memory", "Connection aborted", "Connection refused", "Not connected", "Already connected", "Connection closed", "Initialization error (interapplication manager)", "Bad occurrence", "Wait on unbound occurrence handler", "Occurrence queue overflow", "Datalog type conflict", "Unused", "Unrecognized type (interapplication manager)", "Memory corrupt", "Failed to make temporary DLL", "Old CIN version", "Drag socket not found", "Failed to load drop-object", "Failed to register OLE object", "Failed to release OLE object", "Format specifier type mismatch", "Unknown format specifier", "Too few format specifiers", "Too many format specifiers", "Scan failed", "Newer CIN version", "Error converting to variant", "Runtime menu error", "Password tampered", "Variant attribute not found", "Incompatible variant data type", "Event data is not available", "Event Store is not present", "Occurrence is not found", "Event Queue is not created", "Event info is not available", "Refnum passed is NULL", "Error retrieving Class GUID", "Error retrieving CoClass GUID", "Error retrieving TypeLib GUID.", "Bad built application magic bytes.", "Specific driver is different from the specific driver associated with the Logical Name.", "There is no session opened to the class driver.", "Max Error", "MAX - Error with config objects", "MAX - Error loading configuration", "MAX - Group not supported"]
        # "Current State"
        # "Do not delete, rename, or modify this frame.\n(this is used to capture unhandled states and typos)"
        # "Handle mistyped state name (developer tool)"
        n221 = Format Into String(format string="Software Exception: Unhandled State \"%s\"." ("message"), error in=w676, w671) -> (resulting string=w679:string, error out=w678:errorcluster)  [unwired: 1 in]
        n222 = call <vilib>:"Error Cluster From Error Code.vi"("show call chain? (False)"=TRUE, "error in (no error)"=w678, "error message (\"\")"=w679, "error code (0)"=w680) -> ("error out"=w677:errorcluster)  [unwired: 5 in]
        n223 = call <vilib>:"Add State(s) to Queue__jki_lib_state_machine.vi"("State(s) in (\"\")"=w675) -> ("States Out"=w674:string)  [unwired: 14 in]
      }
      frame "Error Handler" {
        # "Unhandled Error -- Display it"
        # "Handle any errors here.\nYou can also output any states to clean-up after errors occur"
        # "Clear error"
        n224 = call <vilib>:"General Error Handler.vi"("error in (no error)"=w683) -> ()  [unwired: 10 in, 5 out]
        n225 = call <vilib>:"Add State(s) to Queue__jki_lib_state_machine.vi"("State(s) in Front (\"\")"="/* Post Error States", "State(s) in (\"\")"=w687) -> ("States Out"=w686:string)  [unwired: 13 in]
      }
      frame "Exit" {
        # "Do not put any code in this frame.\n(No errors that occur here will be handled.)"
        n226 = call <vilib>:"Add State(s) to Queue__jki_lib_state_machine.vi"("State(s) in (\"\")"=w692) -> ("States Out"=w691:string)  [unwired: 14 in]
      }
      frame "---------- Data ----------" {
        # "Do not put any code in this frame.\n(It is a separator no-op. You can make a copy of this frame to create a new Data frame)"
        n227 = call <vilib>:"Add State(s) to Queue__jki_lib_state_machine.vi"("State(s) in (\"\")"=w696) -> ("States Out"=w695:string)  [unwired: 14 in]
      }
      frame "Data: Initialize" {
        n228 = while {
          tunnel: [w702] -> w697
          stop <- w703 stop-if-true
          w702 = path ""  # Input File Path
          n229 = Wait Until Next ms Multiple(millisecond multiple=u32 1000) -> ()  [unwired: 1 out]
          n230 = local read "Start DAQ Loop"() -> (w703:bool)
        }
        n231 = Bundle("Input File Path"=w697) -> (w699:cluster{"Input File Path":path})  [unwired: 1 in]
        n232 = call <vilib>:"Add State(s) to Queue__jki_lib_state_machine.vi"("State(s) in (\"\")"=w701) -> ("States Out"=w700:string)  [unwired: 14 in]
      }
      frame "---------- Collect Data ----------" {
        n233 = call <vilib>:"Add State(s) to Queue__jki_lib_state_machine.vi"("State(s) in (\"\")"=w708) -> ("States Out"=w707:string)  [unwired: 14 in]
      }
      frame "Save Data" {
        n234 = Dequeue Element(queue=w718, error in (no error)=w717) -> (element=w715:string[], timed out?=w714:bool, error out=w716:errorcluster)  [unwired: 1 in, 1 out]
        n235 = Unbundle By Name(w712) -> ("Input File Path"=w711:path)
        n236 = Equal?(x=w711, y=path "" ("Input File Path")) -> (x = y?=w713:bool)
        n237 = Or(x=w714, y=w713) -> (x .or. y?=w709:bool)
        n238 = case shown="False" w709 {
          tunnel: w712 -> [w724 _]
          tunnel: w716 -> [w722 _]
          tunnel: w715 -> [w721 _]
          frame False {
            n239 = Unbundle By Name(w724) -> ("Input File Path"=w723:path)
            n240 = call-poly <vilib>:"Write Delimited Spreadsheet.vi"("file path (dialog if empty)"=w723, "1D data"=w721, "append to file? (new file:F)"=TRUE, "error in (no error)"=w722, "delimiter (\\t)"="," ("delimiter (\\t)")) -> ()  [unwired: 9 in, 2 out]
          }
          frame True {
          }
        }
        n241 = call <vilib>:"Add State(s) to Queue__jki_lib_state_machine.vi"("State(s) in (\"\")"=w720) -> ("States Out"=w719:string)  [unwired: 14 in]
      }
      frame "Check Exit" {
        n242 = local read "Exit App"() -> (w727:bool)
        n243 = case shown="False" w727 {
          tunnel: ["" ("State(s) in Front (\"\")") "Exit" ("State(s) in Front (\"\")")] -> w728
          frame False {
          }
          frame True {
          }
        }
        n244 = call <vilib>:"Add State(s) to Queue__jki_lib_state_machine.vi"("State(s) in Front (\"\")"=w728, "State(s) in (\"\")"=w732) -> ("States Out"=w731:string)  [unwired: 13 in]
      }
    }
    n245 = local read "Turn on Text Debug Array"() -> (w601:bool)
    n246 = case shown="True" w601 {
      tunnel: w602 -> [_ w619]
      tunnel: [w616 w618] -> w603
      tunnel: w604 -> [w616 w617]
      frame False {
      }
      frame True {
        n247 = Build Array (concatenate)(w617, w619) -> (w618:string[])
        "Debug Save Array" <- w618
      }
    }
  }
  n248 = Release Queue(queue=w5, error in (no error)=w4) -> (error out=w3:errorcluster)  [unwired: 1 in, 2 out]
  n249 = local read "Use GEA Inverter Output"() -> (w12:bool)
  n250 = call "GEA2 Stop.vi"("GEA2 Reference Out"=w20, "Error In"=w3) -> ("Error Out"=w15:errorcluster)  [unwired: 13 in]
  n251 = case shown="False" w12 {
    tunnel: w3 -> [w735 w738]
    tunnel: w16 -> [_ w737]
    tunnel: [w735 w736] -> w14
    frame False {
    }
    frame True {
      n252 = call "GEA2 Stop.vi"("GEA2 Reference Out"=w737, "Error In"=w738) -> ("Error Out"=w736:errorcluster)  [unwired: 13 in]
    }
  }
  n253 = Merge Errors(w15, w14) -> (→"Error Out":errorcluster)
